vi "Parse Raw Payload Frame.vi"(10 "Data":u8[](array[numeric]) format="%.0x") -> (0 "UDPsrcPort":u16=1, 1 "UDPdstPort":u16=1, 2 "VL Id":u16=60, 3 "Payload":u8[](array[numeric]), 5 "Frame Configuration":T1={"domainID"=1, "sideID"=1, "locationID"=1, "interfaceID"=1, "partitionID"=1} {"interfaceID" format="%.0b"})   [LabVIEW 2020]
uses:
  <instrlib>/AIM GmbH/_AIM 664/_controls/queue_data_full.ctl
  <instrlib>/AIM GmbH/_AIM 664/helpers/EthFrameManagement/EthFrameManagement.lvlib
  <instrlib>/AIM GmbH/_AIM 664/AIM664LV.lvlib
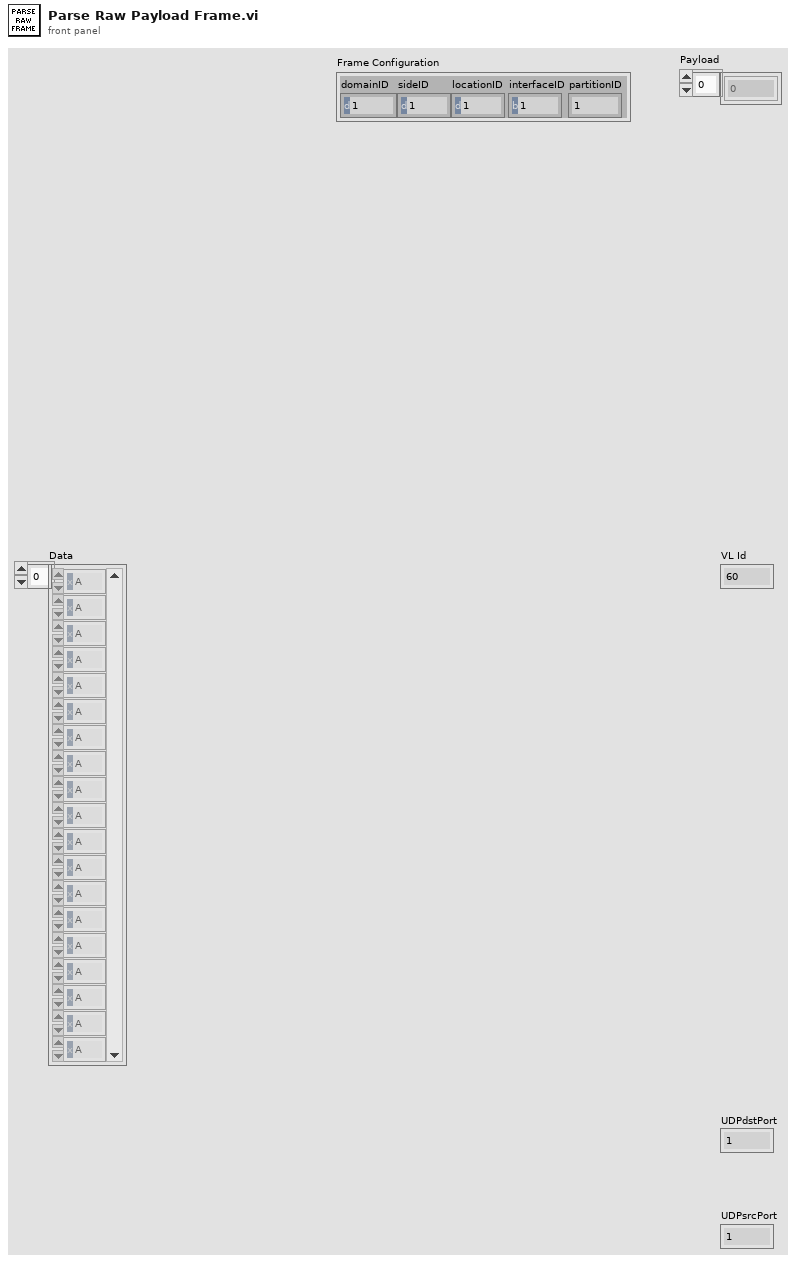
[diagram p1: front panel]
types:
  T1 = typedef "AIM664LV.lvlib/queue_data_full.ctl" = cluster{"domainID":u8, "sideID":u8, "locationID":u8, "interfaceID":u8, "partitionID":u8}
  T2 = typedef "EthFrameManagement.lvlib/ehternetFrame_type.ctl" = cluster{"Dest MAC":u8[], "Src MAC":u8[], "EtherType":u16}
  T3 = typedef "EthFrameManagement.lvlib/IPFrame_type.ctl" = cluster{"Version":u8, "IHL":u8, "ToS":u8, "Length":u16, "ID":u16, "CtlFlags":u8, "FragOffset":u16, "TTL":u8, "Protocol":u8, "Checksum":u16, "Source IP":u32, "Dest IP":u32}
  T4 = typedef "EthFrameManagement.lvlib/UDPFrame_type.ctl" = cluster{"Source Port":u16, "Dest Port":u16, "Lenght":u16, "Checksum":u16}
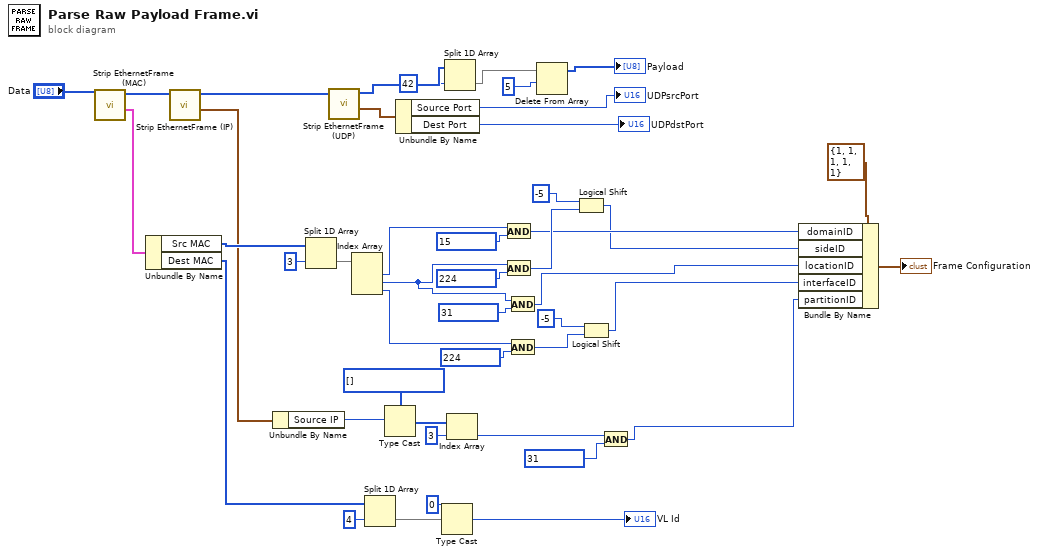
[diagram p0: block diagram]
diagram:
  n1 = call <instrlib>:"Strip EthernetFrame (MAC).vi"("Ethernet Frame In"="Data") -> ("Ethernet header"=w42:T2, "Ethernet Frame Out"=w44:u8[])  [unwired: 7 in, 2 out]
  n2 = Unbundle By Name(w42) -> ("Src MAC"=w8:u8[], "Dest MAC"=w40:u8[])
  n3 = call <instrlib>:"Strip EthernetFrame (IP).vi"("Frame In"=w44) -> ("IP header"=w2:T3, "Frame Out"=w43:u8[])  [unwired: 7 in, 2 out]
  n4 = Unbundle By Name(w2) -> ("Source IP"=w1:u32)
  n5 = Split 1D Array(array=w8, index=3) -> (second subarray=w27:u8[])  [unwired: 1 out]
  n6 = call <instrlib>:"Strip EthernetFrame (UDP).vi"("Ethernet Frame In"=w43) -> ("UDP header"=w41:T4, "Ethernet Frame Out"=w35:u8[])  [unwired: 7 in, 2 out]
  n7 = Index Array(array=w27) -> (element #1=w25:u8, element #2=w23:u8, element #3=w20:u8)  [unwired: 3 in]
  n8 = Split 1D Array(array=w40, index=4) -> (second subarray=w37:u8[])  [unwired: 1 out]
  n9 = Type Cast(type=u8[] [] ("MAC-src"), x=w1) -> (*(type *) &x=w14:u8[])
  n10 = Unbundle By Name(w41) -> ("Source Port"=→"UDPsrcPort":u16, "Dest Port"=→"UDPdstPort":u16)
  n11 = Type Cast(type=u16 0 ("VL Id 2"), x=w37) -> (*(type *) &x=→"VL Id":u16)
  n12 = Split 1D Array(array=w35, index=42) -> (second subarray=w32:u8[])  [unwired: 1 out]
  n13 = Index Array(array=w14, index=3) -> (element=w11:u8)
  n14 = And(x=w25, y=u8 15) -> (x .and. y?=w6:u8)
  n15 = And(x=w23, y=u8 224) -> (x .and. y?=w18:u8)
  n16 = And(x=w23, y=u8 31) -> (x .and. y?=w4:u8)
  n17 = And(x=w20, y=u8 224) -> (x .and. y?=w16:u8)
  n18 = Delete From Array(array=w32, length=5 ("index")) -> (array with subset deleted=→"Payload":u8[])  [unwired: 1 in, 1 out]
  n19 = Logical Shift(y=i16 -5, x=w18) -> (x << y=w5:u8)
  n20 = Logical Shift(y=i16 -5, x=w16) -> (x << y=w3:u8)
  n21 = And(x=w11, y=u8 31) -> (x .and. y?=w7:u8)
  n22 = Bundle By Name(cluster=T1 {"domainID"=1, "sideID"=1, "locationID"=1, "interfaceID"=1, "partitionID"=1} ("Frame Configuration"), "domainID"=w6, "sideID"=w5, "locationID"=w4, "interfaceID"=w3, "partitionID"=w7) -> (→"Frame Configuration":T1)
